vi "simulacion_Tren_Masas.vi"() -> ()   [LabVIEW 2017]
uses:
  <vilib>/addons/Control Design/_Model Construction/Data Typedefs.llb/CD Variables.ctl
  <vilib>/Simulation/Scripting/Companion Diagram/SimConfigNode/SimParams.ctl
  <vilib>/Simulation/Scripting/Companion Diagram/SimConfigNode/_simSolvers.ctl
  <vilib>/Simulation/Implementation/Shared/SIMSCR Execution Mode.ctl
  <vilib>/Simulation/Param Hierarchy/Typedefs/SIMPH Param Control Actions.ctl
  <vilib>/Simulation/Implementation/Shared/NILVSim_ParamChanged.vi
  <vilib>/Simulation/Implementation/Shared/NILVSIM_BeginStep.vi
  <vilib>/Simulation/DataSources/Implementation/NILVSim Step.llb/SIM Step (scalar).vi
  <vilib>/Simulation/Utility/Implementation/SIM Halt.vi
  <vilib>/Simulation/ContinuousLinear/Implementation/NILVSim State Space.llb/SIM State Space Distributor (SISO CD).vi
  <vilib>/Simulation/ContinuousLinear/Implementation/NILVSim State Space.llb/SIM State Space Collector (SISO CD).vi
  <vilib>/Simulation/SignalDisplay/Implementation/NILVSim Time Waveform.llb/SIM Time Waveform (scalar).vi
  <vilib>/Simulation/Implementation/Shared/NILVSim_Manager.vi
  <vilib>/Utility/error.llb/Clear Errors.vi
  <vilib>/Simulation/Implementation/Shared/NILVSim_FinalizeModel.vi
  <vilib>/addons/Control Design/_Model Construction/Model Creation.llb/Model Creation SubVI/cd_Create Symbolic State Space Model.vi
  <vilib>/addons/Control Design/_Utility/Model Viewer.llb/Model Viewer SubVI/cd_Draw State-Space Equation (SS).vi
  <vilib>/Simulation/Implementation/Shared/SIM Unbundle Sim Info.vi
  <vilib>/Simulation/Implementation/Shared/NILVSim_Initialize.vi
  <vilib>/Simulation/Utility/Implementation/NILVSim Get Time and IsAcceptedStep.vi
  <vilib>/Simulation/Implementation/Shared/SIMSH Read Queue.vi
  <vilib>/Simulation/Implementation/Shared/NILVSim_GetModelError.vi
  <vilib>/Simulation/Implementation/Shared/SIM Bundle Sim Info.vi
  <vilib>/Simulation/Scripting/Companion Diagram/SimConfigNode/SimDog.xnode
  <vilib>/Simulation/Implementation/XNodeFramework/SimXNode/SimX.xnode
  <vilib>/addons/Control Design/_Model Construction/NI_LinSys_Model Creation.lvlib
  <vilib>/addons/Control Design/_Utility/NI_CD_Model Viewer.lvlib
  <vilib>/addons/Control Design/_Model Construction/Model Typedefs.llb/CD General Elements.ctl
  <vilib>/addons/Control Design/_Model Construction/NI_LinSys_Model Typedefs.lvlib
  <vilib>/addons/Control Design/_Model Construction/Model Typedefs.llb/CD State Space Model (MIMO).ctl
  <vilib>/Simulation/ContinuousLinear/Implementation/NILVSim State Space.llb/SIM State Space (SISO CD).vi
  <vilib>/Simulation/Implementation/Shared/NI_SIM_Implementation.lvlib
  <vilib>/addons/Control Design/_Model Construction/NI_LinSys_Data Typedefs.lvlib
panel:
  out "Waveform Chart":waveform(dbl)(graph)
  in  "Halt?":bool
  out "Equation":picture
  in  "Variables":T1=[{"Name"="k1", " Value"=1.0}, {"Name"="k2", " Value"=1.0}, {"Name"="k3", " Value"=1.0}, {"Name"="b1", " Value"=1.0}, {"Name"="b2", " Value"=1.0}, {"Name"="b3", " Value"=1.0}, {"Name"="m1", " Value"=1.0}, {"Name"="m2", " Value"=1.0}, {"Name"="m3", " Value"=1.0}] {"Value" format="%.2f"}
  in  "b3":dbl=1.0
  in  "b3":dbl=1.0
  in  "b1":dbl=1.0
  in  "k3":dbl=1.0
  in  "k2":dbl=1.0
  in  "k1":dbl=1.0
  in  "m3":dbl=1.0
  in  "m2":dbl=1.0
  in  "m1":dbl=1.0
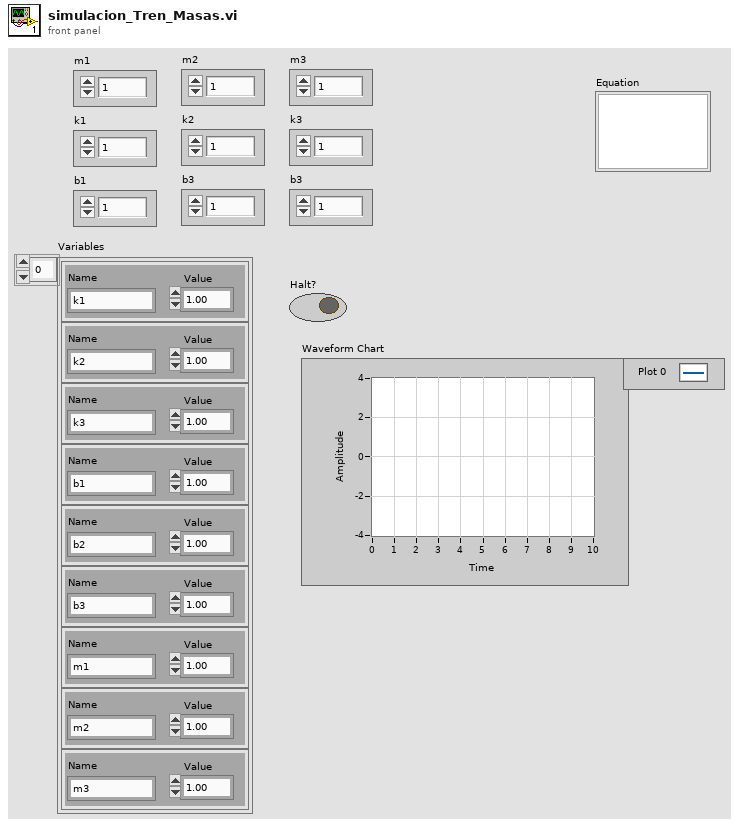
[diagram p1: front panel]
types:
  T1 = typedef "NI_LinSys_Data Typedefs.lvlib/CD Variables.ctl" = cluster{"Name":string, " Value":dbl}[]
  T2 = typedef "NI_LinSys_Model Typedefs.lvlib/CD State Space Model (MIMO).ctl" = cluster{"properties":T3, "A":dbl[][], "B":dbl[][], "C":dbl[][], "D":dbl[][], "StateNames":string[], "Transport Delay":dbl[][]}
  T3 = typedef "NI_LinSys_Model Typedefs.lvlib/CD General Elements.ctl" = cluster{"Model name":string, "Input names":string[], "Output names":string[], "Input Delays":dbl[], "Output Delays":dbl[], "Sampling Time":dbl, "Notes":string}
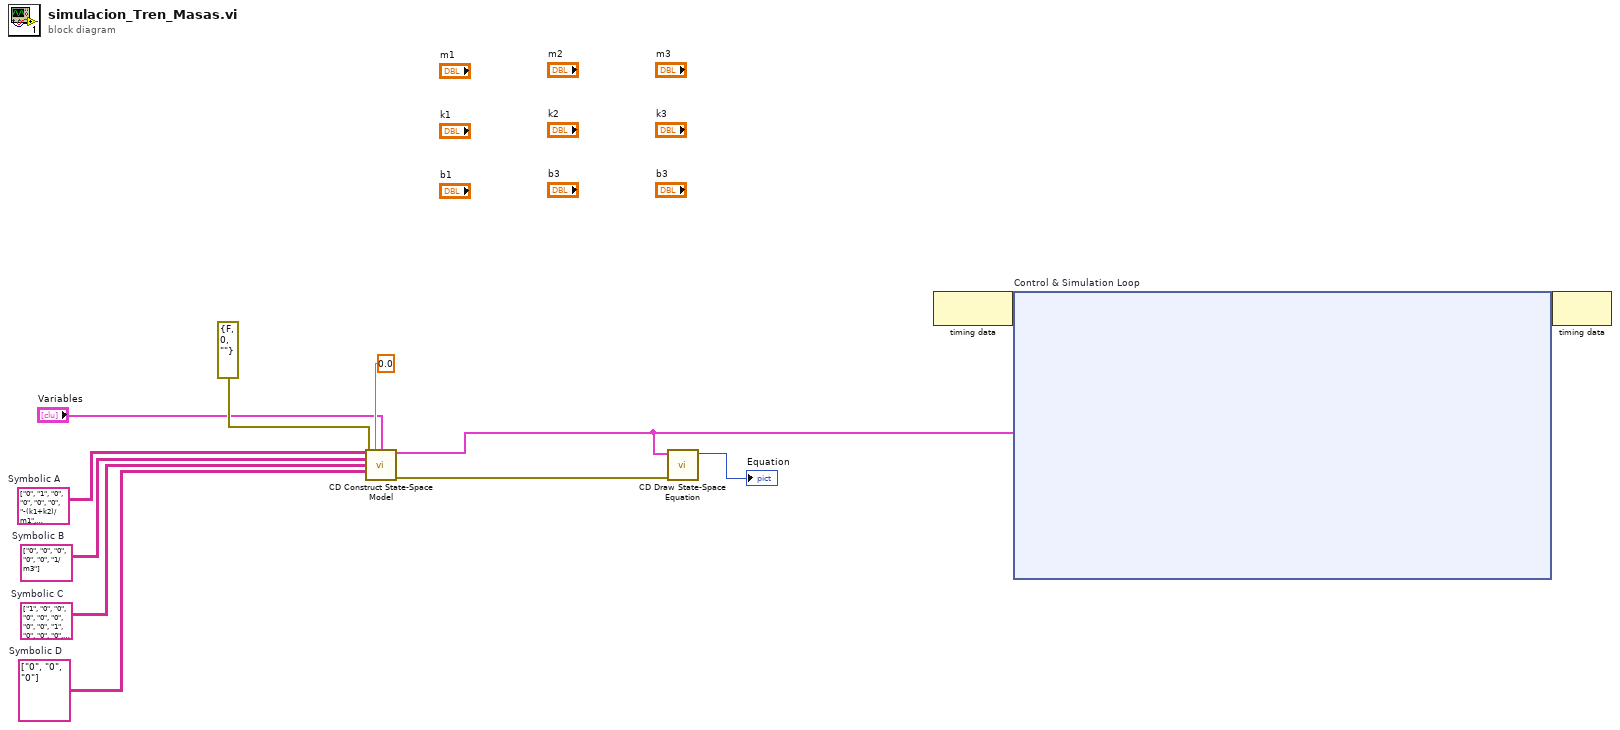
[diagram p0: block diagram]
diagram:
  w2 = string[][] [["1", "0", "0", "0", "0", "0"], ["0", "0", "1", "0", "0", "0"], ["0", "0", "0", "0", "1", "0"]]  # Symbolic C
  w1 = string[][] [["0"], ["0"], ["0"]]  # Symbolic D
  w3 = string[][] [["0"], ["0"], ["0"], ["0"], ["0"], ["1/m3"]]  # Symbolic B
  w4 = string[][] [["0", "1", "0", "0", "0", "0"], ["-(k1+k2)/m1", "-(b1+b2)/m1", "k2/m1", "b2/m1", "0", "0"], ["0", "0", "0", "1", "0", "0"], ["k2/m2", "b2/m2", "-(k2+k3)/m2", "-(b2+b3)/m2", "k3/m2", "b3/m2"], ["0", "0", "0", "0", "0", "1"], ["0", "0", "k3/m3", "b3/m3", "-k3/m3", "-b3/m3"]]  # Symbolic A
  n1 = call-poly <vilib>:"CD Construct State-Space Model.vi"("Symbolic A"=w4, "Sampling Time (s)"=0.0, "Symbolic B"=w3, "Symbolic C"=w2, "Symbolic D"=w1, "error in (no error)"=errorcluster {"status"=FALSE, "code"=0, "source"=""}, "Variables"="Variables") -> ("State Space Model"=w7:T2, "error out"=w6:errorcluster)  [unwired: 7 in]
  n2 = call-poly <vilib>:"CD Draw State-Space Equation.vi"("error in (no error)"=w6, "State-Space Model"=w7) -> ("Equation"=→"Equation":picture)  [unwired: 7 in, 2 out]
  n3 = node-c288() -> (w12:variant)  [unwired: 1 in]
  n4 = node-c254 "Control & Simulation Loop"(w12, w7) -> (w11:variant)
  n5 = node-c288(w11) -> ()  [unwired: 1 out]
